vi "From JSON Tree.vi"(8 "error in (no error)":errorcluster, 10 "JSON in":refnum<class "JSON Datatype.lvclass">, 11 "Request in":refnum<class "Request.lvclass">) -> (0 "error out":errorcluster, 3 "Request out":refnum<class "Request.lvclass">)   [LabVIEW 2015, in "Request.lvclass"]
uses:
  Request.lvclass
  <vilib>/National Instruments/JSON Support for LabVIEW/JSON Data Classes/JSON Datatype/JSON Datatype.lvclass
  params/params.lvclass
  id/id.lvclass
  Request.lvclass/Request.ctl
  <vilib>/National Instruments/JSON Support for LabVIEW/JSON Data Classes/JSON Datatype/To More Specific Type (Object).vi
  <vilib>/National Instruments/JSON Support for LabVIEW/JSON Data Classes/JSON Object/Get Value (String Value).vi
  <vilib>/National Instruments/JSON Support for LabVIEW/JSON Data Classes/JSON Object/Get Value (JSON).vi
  <vilib>/National Instruments/JSON Support for LabVIEW/JSON Data Classes/JSON Object/JSON Object.lvclass
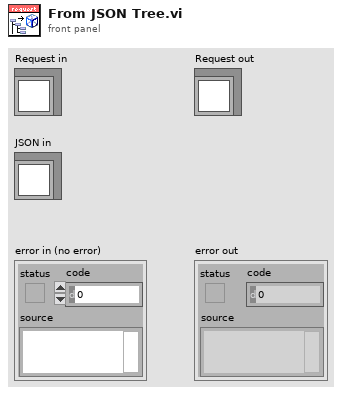
[diagram p1: front panel]
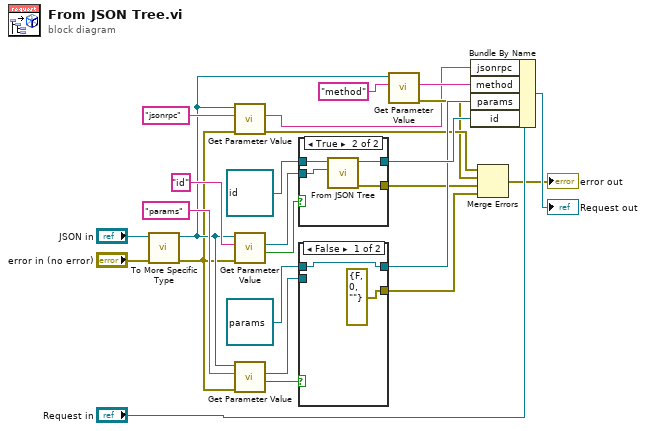
[diagram p0: block diagram]
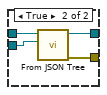
[diagram p2: hidden frame]
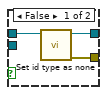
[diagram p3: hidden frame]
diagram:
  n1 = call-poly <vilib>:"To More Specific Type.vi"("error in (no error)"="error in (no error)", "JSON Datatype in"="JSON in") -> ("error out"=w6:errorcluster, "JSON Datatype out"=w8:refnum<class "JSON Object.lvclass">)  [unwired: 8 in]
  n2 = call-poly <vilib>:"Get Parameter Value.vi"("error in (no error)"=w6, "key"="jsonrpc" ("Parameter Name"), "JSON Object in"=w8) -> ("error out"=w11:errorcluster, "value"=w1:string)  [unwired: 6 in, 1 out]
  n3 = call-poly <vilib>:"Get Parameter Value.vi"("error in (no error)"=w6, "key"="id" ("Parameter Name"), "JSON Object in"=w8) -> ("found"=w3:bool, "value"=w4:refnum<class "JSON Datatype.lvclass">)  [unwired: 6 in, 1 out]
  n4 = call-poly <vilib>:"Get Parameter Value.vi"("error in (no error)"=w6, "key"="params" ("Parameter Name"), "JSON Object in"=w8) -> ("found"=w2:bool, "value"=w5:refnum<class "JSON Datatype.lvclass">)  [unwired: 6 in, 1 out]
  n5 = case shown="True" w3 {
    tunnel: refnum<class "id.lvclass"> refnum ("id.lvclass") -> [w28 w32]
    tunnel: w4 -> [_ w31]
    tunnel: [w27 w30] -> w22
    tunnel: [w26 w29] -> w19
    frame False {
      n6 = call-dynamic "Set id type as none.vi"("id in"=w28) -> ("error out"=w26:errorcluster, "id out"=w27:refnum<class "id.lvclass">)  [unwired: 9 in]
    }
    frame True {
      n7 = call-dynamic "From JSON Tree.vi"("JSON in"=w31, "id in"=w32) -> ("error out"=w29:errorcluster, "id out"=w30:refnum<class "id.lvclass">)  [unwired: 8 in]
    }
  }
  n8 = case shown="False" w2 {
    tunnel: refnum<class "params.lvclass"> refnum ("params.lvclass") -> [w34 w38]
    tunnel: w5 -> [_ w37]
    tunnel: [w34 w36] -> w20
    tunnel: [errorcluster {"status"=FALSE, "code"=0, "source"=""} ("error out") w35] -> w12
    frame False {
    }
    frame True {
      n9 = call-dynamic "From JSON Tree.vi"("JSON in"=w37, "params in"=w38) -> ("error out"=w35:errorcluster, "params out"=w36:refnum<class "params.lvclass">)  [unwired: 8 in]
    }
  }
  n10 = call-poly <vilib>:"Get Parameter Value.vi"("key"="method" ("Parameter Name"), "JSON Object in"=w8) -> ("error out"=w10:errorcluster, "value"=w15:string)  [unwired: 7 in, 1 out]
  n11 = Bundle By Name(cluster="Request in", "jsonrpc"=w1, "method"=w15, "params"=w20, "id"=w22) -> (→"Request out":refnum<class "Request.lvclass">)
  n12 = Merge Errors(w11, w10, w19, w12) -> (→"error out":errorcluster)
